vi "PH_ForceSensor.set GUI for first time.vi"(0 "VI in":refnum<vi>, 5 "error in (no error)":errorcluster) -> (14 "VI out":refnum<vi>, 19 "error out":errorcluster)   [LabVIEW 2014, in "PH_ForceSensor.lvlib"]
uses:
  PH_ForceSensor.lvlib
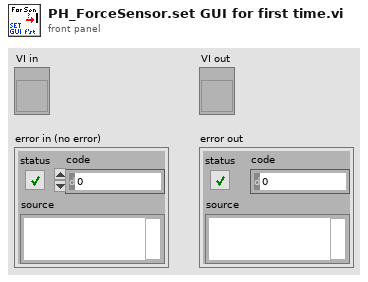
[diagram p1: front panel]
types:
  T1 = typedef "PH_ForceSensor.lvlib/PH_ForceSensor.i attribute.ctl" = cluster{"GUI Refs":T2, "Rawvalues":T3, "Offsets [µV]":T3, "Scalings [mV/V]":T3, "Forces [N]":T3, "Supply Voltage [V]":dbl, "Full Force [N]":dbl, "Ranges [N]":cluster{"Low Energy":cluster{"Upper Limit":dbl, "Lower Limit":dbl}, "High Energy":cluster{"Upper Limit":dbl, "Lower Limit":dbl}}}
  T2 = typedef "PH_ForceSensor.lvlib/PH_ForceSensor.GUI Refs.ctl" = cluster{"Delete":refnum<vi>, "Rawvalues":refnum<vi>, "Offsets [µV]":refnum<vi>, "Sensor Values [µV]":refnum<vi>, "Scalings [mV/V]":refnum<vi>, "Supply Voltage [V]":refnum<vi>, "Full Force [N]":refnum<vi>, "Forces [N]":refnum<vi>, "Graph Differential Forces":refnum<vi>, "Graph Absolute Forces":refnum<vi>, "Ranges [N]":refnum<vi>}
  T3 = typedef "PH_ForceSensor.lvlib/PH_ForceSensor.Dataset.ctl" = cluster{"top front":dbl, "top back":dbl, "bottom front":dbl, "bottom back":dbl}
  T4 = cluster{"Low Energy":cluster{"Upper Limit":dbl, "Lower Limit":dbl}, "High Energy":cluster{"Upper Limit":dbl, "Lower Limit":dbl}}
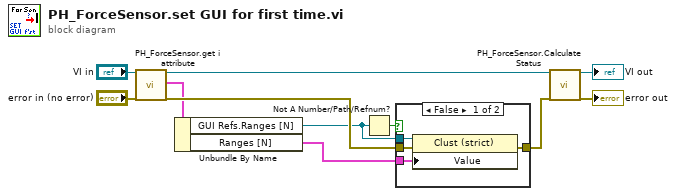
[diagram p0: block diagram]
diagram:
  n1 = call "PH_ForceSensor.get i attribute.vi"("i ref in"="VI in", "error in (no error)"="error in (no error)") -> ("i ref out"=w2:refnum<vi>, "i attribute"=w8:T1, "error out"=w10:errorcluster)  [unwired: 15 in]
  n2 = Unbundle By Name(w8) -> ("GUI Refs.Ranges [N]"=w4:refnum<vi>, "Ranges [N]"=w6:T4)
  n3 = Not A Number/Path/Refnum?(number/path/refnum=w4) -> (NaN/Path/Refnum?=w5:bool)
  n4 = case shown="False" w5 {
    tunnel: w10 -> [w15 w16]
    tunnel: [w14 w16] -> w7
    tunnel: w4 -> [w13 _]
    tunnel: w6 -> [w12 _]
    frame False {
      n5 = property class="Clust (strict)"(reference=w13, error in=w15, "Value"=w12) -> (error out=w14:errorcluster)  [unwired: 1 out]
    }
    frame True {
    }
  }
  n6 = call "PH_ForceSensor.Calculate Status.vi"("VI in"=w2, "error in"=w7) -> ("VI out"=→"VI out":refnum<vi>, "error out"=→"error out":errorcluster)  [unwired: 16 in]
